vi "InitDrivebase.vi"   [LabVIEW 2019]
doc: "This VI initializes devices related directly to the drive subsystem."
uses:
  <vilib>/Rock Robotics/WPI/Solenoid/WPI_SolenoidChannel.ctl
  <vilib>/Rock Robotics/WPI/ThirdParty/Phoenix-LabVIEW/Motor Controller/Controls/CTRE_Phoenix_MotorControl_SupplyCurrentLimitConfiguration.ctl
  <vilib>/Rock Robotics/WPI/ThirdParty/Phoenix-LabVIEW/Motor Controller/Controls/CTRE_Phoenix_MotorControl_FeedbackDevice_TalonFX.ctl
  <vilib>/Rock Robotics/WPI/ThirdParty/Phoenix-LabVIEW/Motor Controller/Controls/CTRE_Phoenix_MotorControl_TalonFXInvertType.ctl
  <vilib>/Rock Robotics/WPI/ThirdParty/Phoenix-LabVIEW/Motor Controller/Controls/CTRE_Phoenix_MotorControl_NeutralMode.ctl
  <vilib>/Rock Robotics/WPI/Solenoid/WPI_SolenoidOpenDouble.vi
  refnums.vi
types:
  T1 = typedef "WPI_SolenoidChannel.ctl" = enum8{"Solenoid 0", "Solenoid 1", "Solenoid 2", "Solenoid 3", "Solenoid 4", "Solenoid 5", "Solenoid 6", "Solenoid 7", "Invalid"}
  T2 = typedef "CTRE_Phoenix_MotorControl_TalonFXInvertType.ctl" = enum16{"Counter-Clockwise", "Clockwise"}
  T3 = typedef "CTRE_Phoenix_MotorControl_FeedbackDevice_TalonFX.ctl" = i8
  T4 = typedef "CTRE_Phoenix_MotorControl_SupplyCurrentLimitConfiguration.ctl" = cluster{"Enable?":bool, "Current Limit":dbl, "Threshold Current":dbl, "Threshold Time":dbl}
  T5 = typedef "CTRE_Phoenix_MotorControl_NeutralMode.ctl" = enum8{"EEPROMSetting", "Override to Coast", "Override to Brake"}
  T6 = typedef "WPI_MotorControlDeviceRef.ctl" = cluster{"DeviceStatus":errorcluster, "Type":T7, "PWM":cluster{"PWM Channel":T8, "DeadBand":T9}, "CAN":cluster{"Device Number":u8, "SetOutput VI Ref":variant, "GetOutput VI Ref":variant, "Enable VI Ref":variant, "Disable VI Ref":variant, "Data":variant}, "Invert":bool, "DIO PWM":cluster{"PWM \"Enable\" Channel":T8, "DIOChannel":T10, "PWM Rate":dbl}}
  T7 = typedef "WPI_MotorControlType.ctl" = enum16{"PWM", "CAN", "DIO PWM"}
  T8 = typedef "FPGA_DIOPWMChannel.ctl" = enum8{"PWM 0", "PWM 1", "PWM 2", "PWM 3", "PWM 4", "PWM 5", "PWM 6", "PWM 7", "PWM 8", "PWM 9", "PWM MXP 0", "PWM MXP 1", "PWM MXP 2", "PWM MXP 3", "PWM MXP 4", "PWM MXP 5", "PWM MXP 6", "PWM MXP 7", "PWM MXP 8", "PWM MXP 9", "Invalid"}
  T9 = typedef "WPI_PWMDeadband.ctl" = cluster{"Name":string, "maxPositivePwm":i32, "minPositivePwm":i32, "centerPwm":i32, "maxNegativePwm":i32, "minNegativePwm":i32, "angularRange":u16}
  T10 = typedef "FPGA_DIOChannel.ctl" = enum8{"DIO 0", "DIO 1", "DIO 2", "DIO 3", "DIO 4", "DIO 5", "DIO 6", "DIO 7", "DIO 8", "DIO 9", "DIO MXP 0", "DIO MXP 1", "DIO MXP 2", "DIO MXP 3", "DIO MXP 4", "DIO MXP 5", "DIO MXP 6", "DIO MXP 7", "DIO MXP 8", "DIO MXP 9", "DIO MXP 10", "DIO MXP 11", "DIO MXP 12", "DIO MXP 13", "DIO MXP 14", "DIO MXP 15", "SPI Port CS1", "SPI Port CS2", "SPI Port CS3", "SPI Port MISO", "SPI Port MOSI", "Invalid"}
  T11 = typedef "WPI_SolenoidDevRef.ctl" = cluster{"DevStatus":errorcluster, "Pneumatics Control Module":u8, "Forward Solenoid Channel":T1, "Reverse Solenoid Channel":T1}
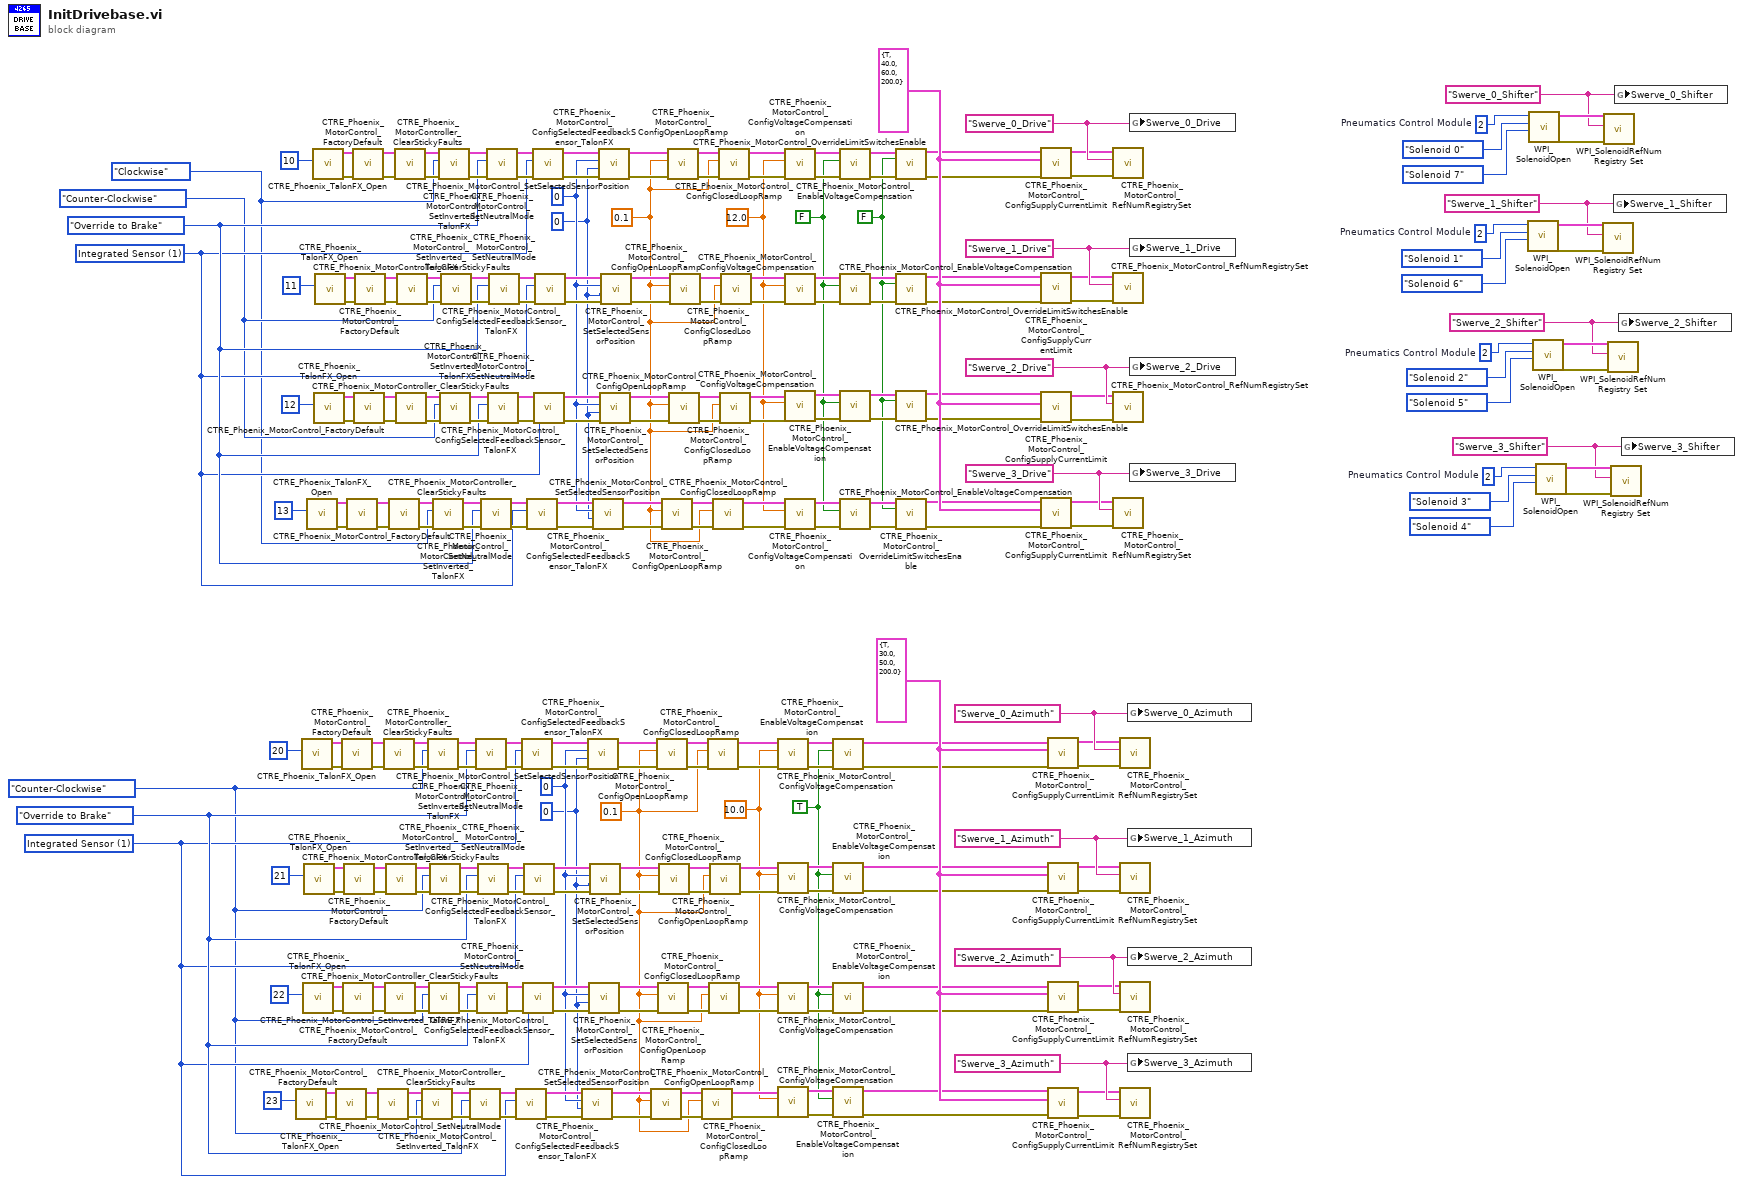
[diagram p0: block diagram]
diagram:
  w1 = FALSE ("Override Limit Switch Enable?")
  w19 = "Swerve_0_Shifter" ("refnum name")
  w24 = u8 2  # Pneumatics Control Module
  w25 = "Swerve_1_Shifter" ("refnum name")
  w30 = u8 2  # Pneumatics Control Module
  w31 = "Swerve_2_Shifter" ("refnum name")
  w36 = u8 2  # Pneumatics Control Module
  w37 = CTRE_Phoenix_MotorControl_TalonFXInvertType."Clockwise" ("Invert Type")
  w39 = TRUE ("Enable Voltage Compensation?")
  w40 = 10.0 ("Saturation Voltage")
  w41 = FALSE ("Enable Voltage Compensation?")
  w42 = 12.0 ("Saturation Voltage")
  w83 = T3 1 items=["Integrated Sensor"=1, "Sensor Sum (S0 + S1)"=9, "Sensor Difference (D0 - D1)"=10, "Remote Source 0"=11, "Remote Source 1"=12, "None"=14, "Software Emulated"=15] ("Talon FX Feedback Device")
  w88 = T4 {"Enable?"=TRUE, "Current Limit"=30.0, "Threshold Current"=50.0, "Threshold Time"=200.0} ("Supply Current Limit Configuration")
  w84 = 0.1 ("secondsFromNeutralToFull")
  w85 = u32 0 ("pidLoopIdx")
  w86 = 0 ("New Sensor Position")
  w87 = CTRE_Phoenix_MotorControl_NeutralMode."Override to Brake" ("Motor Control Neutral Mode")
  w18 = CTRE_Phoenix_MotorControl_TalonFXInvertType."Counter-Clockwise" ("Invert Type")
  w104 = "Swerve_0_Azimuth" ("refnum name")
  w124 = "Swerve_1_Azimuth" ("refnum name")
  w144 = "Swerve_2_Azimuth" ("refnum name")
  w164 = "Swerve_3_Azimuth" ("refnum name")
  w172 = T3 1 items=["Integrated Sensor"=1, "Sensor Sum (S0 + S1)"=9, "Sensor Difference (D0 - D1)"=10, "Remote Source 0"=11, "Remote Source 1"=12, "None"=14, "Software Emulated"=15] ("Talon FX Feedback Device")
  w174 = T4 {"Enable?"=TRUE, "Current Limit"=40.0, "Threshold Current"=60.0, "Threshold Time"=200.0} ("Supply Current Limit Configuration")
  w169 = 0.1 ("secondsFromNeutralToFull")
  w170 = u32 0 ("pidLoopIdx")
  w171 = 0 ("New Sensor Position")
  w173 = CTRE_Phoenix_MotorControl_NeutralMode."Override to Brake" ("Motor Control Neutral Mode")
  w38 = CTRE_Phoenix_MotorControl_TalonFXInvertType."Counter-Clockwise" ("Invert Type")
  w190 = "Swerve_0_Drive" ("refnum name")
  w210 = "Swerve_1_Drive" ("refnum name")
  w230 = "Swerve_2_Drive" ("refnum name")
  w250 = "Swerve_3_Drive" ("refnum name")
  w255 = "Swerve_3_Shifter" ("refnum name")
  w260 = u8 2  # Pneumatics Control Module
  n1 = call <vilib>:"CTRE_Phoenix_TalonFX_Open.vi"("Device Number"=u8 23 ("Drive 4L")) -> ("error out"=w153:errorcluster, "CAN Talon SRX Ref"=w160:T6)  [unwired: 9 in]
  n2 = call <vilib>:"CTRE_Phoenix_TalonFX_Open.vi"("Device Number"=u8 20 ("Drive 4L")) -> ("error out"=w93:errorcluster, "CAN Talon SRX Ref"=w100:T6)  [unwired: 9 in]
  n3 = call <vilib>:"CTRE_Phoenix_TalonFX_Open.vi"("Device Number"=u8 22 ("Drive 4L")) -> ("error out"=w133:errorcluster, "CAN Talon SRX Ref"=w140:T6)  [unwired: 9 in]
  n4 = call <vilib>:"CTRE_Phoenix_TalonFX_Open.vi"("Device Number"=u8 21 ("Drive 4L")) -> ("error out"=w113:errorcluster, "CAN Talon SRX Ref"=w120:T6)  [unwired: 9 in]
  n5 = call <vilib>:"CTRE_Phoenix_TalonFX_Open.vi"("Device Number"=u8 13 ("Drive 4L")) -> ("error out"=w239:errorcluster, "CAN Talon SRX Ref"=w246:T6)  [unwired: 9 in]
  n6 = call <vilib>:"CTRE_Phoenix_TalonFX_Open.vi"("Device Number"=u8 10 ("Drive 4L")) -> ("error out"=w179:errorcluster, "CAN Talon SRX Ref"=w186:T6)  [unwired: 9 in]
  n7 = call <vilib>:"CTRE_Phoenix_TalonFX_Open.vi"("Device Number"=u8 12 ("Drive 4L")) -> ("error out"=w219:errorcluster, "CAN Talon SRX Ref"=w226:T6)  [unwired: 9 in]
  n8 = call <vilib>:"CTRE_Phoenix_TalonFX_Open.vi"("Device Number"=u8 11 ("Drive 4L")) -> ("error out"=w199:errorcluster, "CAN Talon SRX Ref"=w206:T6)  [unwired: 9 in]
  n9 = call <vilib>:"CTRE_Phoenix_MotorControl_FactoryDefault.vi"("error in"=w153, "PhoenixMotorControlDevRef"=w160) -> ("error out"=w156:errorcluster, "PhoenixMotorControlDevRef"=w157:T6)  [unwired: 8 in]
  n10 = call <vilib>:"CTRE_Phoenix_MotorControl_FactoryDefault.vi"("error in"=w93, "PhoenixMotorControlDevRef"=w100) -> ("error out"=w96:errorcluster, "PhoenixMotorControlDevRef"=w97:T6)  [unwired: 8 in]
  n11 = call <vilib>:"CTRE_Phoenix_MotorControl_FactoryDefault.vi"("error in"=w133, "PhoenixMotorControlDevRef"=w140) -> ("error out"=w136:errorcluster, "PhoenixMotorControlDevRef"=w137:T6)  [unwired: 8 in]
  n12 = call <vilib>:"CTRE_Phoenix_MotorControl_FactoryDefault.vi"("error in"=w113, "PhoenixMotorControlDevRef"=w120) -> ("error out"=w116:errorcluster, "PhoenixMotorControlDevRef"=w117:T6)  [unwired: 8 in]
  n13 = call <vilib>:"CTRE_Phoenix_MotorControl_FactoryDefault.vi"("error in"=w239, "PhoenixMotorControlDevRef"=w246) -> ("error out"=w242:errorcluster, "PhoenixMotorControlDevRef"=w243:T6)  [unwired: 8 in]
  n14 = call <vilib>:"CTRE_Phoenix_MotorControl_FactoryDefault.vi"("error in"=w179, "PhoenixMotorControlDevRef"=w186) -> ("error out"=w182:errorcluster, "PhoenixMotorControlDevRef"=w183:T6)  [unwired: 8 in]
  n15 = call <vilib>:"CTRE_Phoenix_MotorControl_FactoryDefault.vi"("error in"=w219, "PhoenixMotorControlDevRef"=w226) -> ("error out"=w222:errorcluster, "PhoenixMotorControlDevRef"=w223:T6)  [unwired: 8 in]
  n16 = call <vilib>:"CTRE_Phoenix_MotorControl_FactoryDefault.vi"("error in"=w199, "PhoenixMotorControlDevRef"=w206) -> ("error out"=w202:errorcluster, "PhoenixMotorControlDevRef"=w203:T6)  [unwired: 8 in]
  n17 = call <vilib>:"CTRE_Phoenix_MotorController_ClearStickyFaults.vi"("error in"=w156, "PhoenixMotorControlDevRef"=w157) -> ("error out"=w155:errorcluster, "PhoenixMotorControlDevRef"=w154:T6)  [unwired: 8 in]
  n18 = call <vilib>:"CTRE_Phoenix_MotorController_ClearStickyFaults.vi"("error in"=w96, "PhoenixMotorControlDevRef"=w97) -> ("error out"=w95:errorcluster, "PhoenixMotorControlDevRef"=w94:T6)  [unwired: 8 in]
  n19 = call <vilib>:"CTRE_Phoenix_MotorController_ClearStickyFaults.vi"("error in"=w136, "PhoenixMotorControlDevRef"=w137) -> ("error out"=w135:errorcluster, "PhoenixMotorControlDevRef"=w134:T6)  [unwired: 8 in]
  n20 = call <vilib>:"CTRE_Phoenix_MotorController_ClearStickyFaults.vi"("error in"=w116, "PhoenixMotorControlDevRef"=w117) -> ("error out"=w115:errorcluster, "PhoenixMotorControlDevRef"=w114:T6)  [unwired: 8 in]
  n21 = call <vilib>:"CTRE_Phoenix_MotorController_ClearStickyFaults.vi"("error in"=w242, "PhoenixMotorControlDevRef"=w243) -> ("error out"=w241:errorcluster, "PhoenixMotorControlDevRef"=w240:T6)  [unwired: 8 in]
  n22 = call <vilib>:"CTRE_Phoenix_MotorController_ClearStickyFaults.vi"("error in"=w182, "PhoenixMotorControlDevRef"=w183) -> ("error out"=w181:errorcluster, "PhoenixMotorControlDevRef"=w180:T6)  [unwired: 8 in]
  n23 = call <vilib>:"CTRE_Phoenix_MotorController_ClearStickyFaults.vi"("error in"=w222, "PhoenixMotorControlDevRef"=w223) -> ("error out"=w221:errorcluster, "PhoenixMotorControlDevRef"=w220:T6)  [unwired: 8 in]
  n24 = call <vilib>:"CTRE_Phoenix_MotorController_ClearStickyFaults.vi"("error in"=w202, "PhoenixMotorControlDevRef"=w203) -> ("error out"=w201:errorcluster, "PhoenixMotorControlDevRef"=w200:T6)  [unwired: 8 in]
  n25 = call <vilib>:"CTRE_Phoenix_MotorControl_SetInverted_TalonFX.vi"("error in (no error)"=w155, "Invert Type"=w18, "PhoenixMotorControlDevRef"=w154) -> ("error out"=w167:errorcluster, "PhoenixMotorControlDevRef"=w168:T6)  [unwired: 7 in]
  n26 = call <vilib>:"CTRE_Phoenix_MotorControl_SetInverted_TalonFX.vi"("error in (no error)"=w95, "Invert Type"=w18, "PhoenixMotorControlDevRef"=w94) -> ("error out"=w107:errorcluster, "PhoenixMotorControlDevRef"=w108:T6)  [unwired: 7 in]
  n27 = call <vilib>:"CTRE_Phoenix_MotorControl_SetInverted_TalonFX.vi"("error in (no error)"=w135, "Invert Type"=w18, "PhoenixMotorControlDevRef"=w134) -> ("error out"=w147:errorcluster, "PhoenixMotorControlDevRef"=w148:T6)  [unwired: 7 in]
  n28 = call <vilib>:"CTRE_Phoenix_MotorControl_SetInverted_TalonFX.vi"("error in (no error)"=w115, "Invert Type"=w18, "PhoenixMotorControlDevRef"=w114) -> ("error out"=w127:errorcluster, "PhoenixMotorControlDevRef"=w128:T6)  [unwired: 7 in]
  n29 = call <vilib>:"CTRE_Phoenix_MotorControl_SetInverted_TalonFX.vi"("error in (no error)"=w241, "Invert Type"=w37, "PhoenixMotorControlDevRef"=w240) -> ("error out"=w253:errorcluster, "PhoenixMotorControlDevRef"=w254:T6)  [unwired: 7 in]
  n30 = call <vilib>:"CTRE_Phoenix_MotorControl_SetInverted_TalonFX.vi"("error in (no error)"=w181, "Invert Type"=w37, "PhoenixMotorControlDevRef"=w180) -> ("error out"=w193:errorcluster, "PhoenixMotorControlDevRef"=w194:T6)  [unwired: 7 in]
  n31 = call <vilib>:"CTRE_Phoenix_MotorControl_SetInverted_TalonFX.vi"("error in (no error)"=w221, "Invert Type"=w38, "PhoenixMotorControlDevRef"=w220) -> ("error out"=w233:errorcluster, "PhoenixMotorControlDevRef"=w234:T6)  [unwired: 7 in]
  n32 = call <vilib>:"CTRE_Phoenix_MotorControl_SetInverted_TalonFX.vi"("error in (no error)"=w201, "Invert Type"=w38, "PhoenixMotorControlDevRef"=w200) -> ("error out"=w213:errorcluster, "PhoenixMotorControlDevRef"=w214:T6)  [unwired: 7 in]
  n33 = call <vilib>:"CTRE_Phoenix_MotorControl_SetNeutralMode.vi"("error in (no error)"=w167, "Motor Control Neutral Mode"=w87, "PhoenixMotorControlDevRef"=w168) -> ("error out"=w151:errorcluster, "PhoenixMotorControlDevRef"=w152:T6)  [unwired: 7 in]
  n34 = call <vilib>:"CTRE_Phoenix_MotorControl_SetNeutralMode.vi"("error in (no error)"=w107, "Motor Control Neutral Mode"=w87, "PhoenixMotorControlDevRef"=w108) -> ("error out"=w91:errorcluster, "PhoenixMotorControlDevRef"=w92:T6)  [unwired: 7 in]
  n35 = call <vilib>:"CTRE_Phoenix_MotorControl_SetNeutralMode.vi"("error in (no error)"=w147, "Motor Control Neutral Mode"=w87, "PhoenixMotorControlDevRef"=w148) -> ("error out"=w131:errorcluster, "PhoenixMotorControlDevRef"=w132:T6)  [unwired: 7 in]
  n36 = call <vilib>:"CTRE_Phoenix_MotorControl_SetNeutralMode.vi"("error in (no error)"=w127, "Motor Control Neutral Mode"=w87, "PhoenixMotorControlDevRef"=w128) -> ("error out"=w111:errorcluster, "PhoenixMotorControlDevRef"=w112:T6)  [unwired: 7 in]
  n37 = call <vilib>:"CTRE_Phoenix_MotorControl_SetNeutralMode.vi"("error in (no error)"=w253, "Motor Control Neutral Mode"=w173, "PhoenixMotorControlDevRef"=w254) -> ("error out"=w237:errorcluster, "PhoenixMotorControlDevRef"=w238:T6)  [unwired: 7 in]
  n38 = call <vilib>:"CTRE_Phoenix_MotorControl_SetNeutralMode.vi"("error in (no error)"=w193, "Motor Control Neutral Mode"=w173, "PhoenixMotorControlDevRef"=w194) -> ("error out"=w177:errorcluster, "PhoenixMotorControlDevRef"=w178:T6)  [unwired: 7 in]
  n39 = call <vilib>:"CTRE_Phoenix_MotorControl_SetNeutralMode.vi"("error in (no error)"=w233, "Motor Control Neutral Mode"=w173, "PhoenixMotorControlDevRef"=w234) -> ("error out"=w217:errorcluster, "PhoenixMotorControlDevRef"=w218:T6)  [unwired: 7 in]
  n40 = call <vilib>:"CTRE_Phoenix_MotorControl_SetNeutralMode.vi"("error in (no error)"=w213, "Motor Control Neutral Mode"=w173, "PhoenixMotorControlDevRef"=w214) -> ("error out"=w197:errorcluster, "PhoenixMotorControlDevRef"=w198:T6)  [unwired: 7 in]
  n41 = call <vilib>:"CTRE_Phoenix_MotorControl_ConfigSelectedFeedbackSensor_TalonFX.vi"("error in (no error)"=w151, "Talon FX Feedback Device"=w83, "PhoenixMotorControlDevRef"=w152) -> ("error out"=w149:errorcluster, "PhoenixMotorControlDevRef"=w150:T6)  [unwired: 7 in]
  n42 = call <vilib>:"CTRE_Phoenix_MotorControl_ConfigSelectedFeedbackSensor_TalonFX.vi"("error in (no error)"=w91, "Talon FX Feedback Device"=w83, "PhoenixMotorControlDevRef"=w92) -> ("error out"=w89:errorcluster, "PhoenixMotorControlDevRef"=w90:T6)  [unwired: 7 in]
  n43 = call <vilib>:"CTRE_Phoenix_MotorControl_ConfigSelectedFeedbackSensor_TalonFX.vi"("error in (no error)"=w131, "Talon FX Feedback Device"=w83, "PhoenixMotorControlDevRef"=w132) -> ("error out"=w129:errorcluster, "PhoenixMotorControlDevRef"=w130:T6)  [unwired: 7 in]
  n44 = call <vilib>:"CTRE_Phoenix_MotorControl_ConfigSelectedFeedbackSensor_TalonFX.vi"("error in (no error)"=w111, "Talon FX Feedback Device"=w83, "PhoenixMotorControlDevRef"=w112) -> ("error out"=w109:errorcluster, "PhoenixMotorControlDevRef"=w110:T6)  [unwired: 7 in]
  n45 = call <vilib>:"CTRE_Phoenix_MotorControl_ConfigSelectedFeedbackSensor_TalonFX.vi"("error in (no error)"=w237, "Talon FX Feedback Device"=w172, "PhoenixMotorControlDevRef"=w238) -> ("error out"=w235:errorcluster, "PhoenixMotorControlDevRef"=w236:T6)  [unwired: 7 in]
  n46 = call <vilib>:"CTRE_Phoenix_MotorControl_ConfigSelectedFeedbackSensor_TalonFX.vi"("error in (no error)"=w177, "Talon FX Feedback Device"=w172, "PhoenixMotorControlDevRef"=w178) -> ("error out"=w175:errorcluster, "PhoenixMotorControlDevRef"=w176:T6)  [unwired: 7 in]
  n47 = call <vilib>:"CTRE_Phoenix_MotorControl_ConfigSelectedFeedbackSensor_TalonFX.vi"("error in (no error)"=w217, "Talon FX Feedback Device"=w172, "PhoenixMotorControlDevRef"=w218) -> ("error out"=w215:errorcluster, "PhoenixMotorControlDevRef"=w216:T6)  [unwired: 7 in]
  n48 = call <vilib>:"CTRE_Phoenix_MotorControl_ConfigSelectedFeedbackSensor_TalonFX.vi"("error in (no error)"=w197, "Talon FX Feedback Device"=w172, "PhoenixMotorControlDevRef"=w198) -> ("error out"=w195:errorcluster, "PhoenixMotorControlDevRef"=w196:T6)  [unwired: 7 in]
  n49 = call <vilib>:"CTRE_Phoenix_MotorControl_SetSelectedSensorPosition.vi"("error in (no error)"=w149, "pidLoopIdx"=w85, "New Sensor Position"=w86, "PhoenixMotorControlDevRef"=w150) -> ("error out"=w166:errorcluster, "PhoenixMotorControlDevRef"=w165:T6)  [unwired: 6 in]
  n50 = call <vilib>:"CTRE_Phoenix_MotorControl_SetSelectedSensorPosition.vi"("error in (no error)"=w89, "pidLoopIdx"=w85, "New Sensor Position"=w86, "PhoenixMotorControlDevRef"=w90) -> ("error out"=w106:errorcluster, "PhoenixMotorControlDevRef"=w105:T6)  [unwired: 6 in]
  n51 = call <vilib>:"CTRE_Phoenix_MotorControl_SetSelectedSensorPosition.vi"("error in (no error)"=w129, "pidLoopIdx"=w85, "New Sensor Position"=w86, "PhoenixMotorControlDevRef"=w130) -> ("error out"=w146:errorcluster, "PhoenixMotorControlDevRef"=w145:T6)  [unwired: 6 in]
  n52 = call <vilib>:"CTRE_Phoenix_MotorControl_SetSelectedSensorPosition.vi"("error in (no error)"=w109, "pidLoopIdx"=w85, "New Sensor Position"=w86, "PhoenixMotorControlDevRef"=w110) -> ("error out"=w126:errorcluster, "PhoenixMotorControlDevRef"=w125:T6)  [unwired: 6 in]
  n53 = call <vilib>:"CTRE_Phoenix_MotorControl_SetSelectedSensorPosition.vi"("error in (no error)"=w235, "pidLoopIdx"=w170, "New Sensor Position"=w171, "PhoenixMotorControlDevRef"=w236) -> ("error out"=w252:errorcluster, "PhoenixMotorControlDevRef"=w251:T6)  [unwired: 6 in]
  n54 = call <vilib>:"CTRE_Phoenix_MotorControl_SetSelectedSensorPosition.vi"("error in (no error)"=w175, "pidLoopIdx"=w170, "New Sensor Position"=w171, "PhoenixMotorControlDevRef"=w176) -> ("error out"=w192:errorcluster, "PhoenixMotorControlDevRef"=w191:T6)  [unwired: 6 in]
  n55 = call <vilib>:"CTRE_Phoenix_MotorControl_SetSelectedSensorPosition.vi"("error in (no error)"=w215, "pidLoopIdx"=w170, "New Sensor Position"=w171, "PhoenixMotorControlDevRef"=w216) -> ("error out"=w232:errorcluster, "PhoenixMotorControlDevRef"=w231:T6)  [unwired: 6 in]
  n56 = call <vilib>:"CTRE_Phoenix_MotorControl_SetSelectedSensorPosition.vi"("error in (no error)"=w195, "pidLoopIdx"=w170, "New Sensor Position"=w171, "PhoenixMotorControlDevRef"=w196) -> ("error out"=w212:errorcluster, "PhoenixMotorControlDevRef"=w211:T6)  [unwired: 6 in]
  n57 = call <vilib>:"CTRE_Phoenix_MotorControl_ConfigOpenLoopRamp.vi"("error in (no error)"=w166, "secondsFromNeutralToFull"=w84, "PhoenixMotorControlDevRef"=w165) -> ("error out"=w158:errorcluster, "PhoenixMotorControlDevRef"=w159:T6)  [unwired: 7 in]
  n58 = call <vilib>:"CTRE_Phoenix_MotorControl_ConfigOpenLoopRamp.vi"("error in (no error)"=w106, "secondsFromNeutralToFull"=w84, "PhoenixMotorControlDevRef"=w105) -> ("error out"=w98:errorcluster, "PhoenixMotorControlDevRef"=w99:T6)  [unwired: 7 in]
  n59 = call <vilib>:"CTRE_Phoenix_MotorControl_ConfigOpenLoopRamp.vi"("error in (no error)"=w146, "secondsFromNeutralToFull"=w84, "PhoenixMotorControlDevRef"=w145) -> ("error out"=w138:errorcluster, "PhoenixMotorControlDevRef"=w139:T6)  [unwired: 7 in]
  n60 = call <vilib>:"CTRE_Phoenix_MotorControl_ConfigOpenLoopRamp.vi"("error in (no error)"=w126, "secondsFromNeutralToFull"=w84, "PhoenixMotorControlDevRef"=w125) -> ("error out"=w118:errorcluster, "PhoenixMotorControlDevRef"=w119:T6)  [unwired: 7 in]
  n61 = call <vilib>:"CTRE_Phoenix_MotorControl_ConfigOpenLoopRamp.vi"("error in (no error)"=w252, "secondsFromNeutralToFull"=w169, "PhoenixMotorControlDevRef"=w251) -> ("error out"=w244:errorcluster, "PhoenixMotorControlDevRef"=w245:T6)  [unwired: 7 in]
  n62 = call <vilib>:"CTRE_Phoenix_MotorControl_ConfigOpenLoopRamp.vi"("error in (no error)"=w192, "secondsFromNeutralToFull"=w169, "PhoenixMotorControlDevRef"=w191) -> ("error out"=w184:errorcluster, "PhoenixMotorControlDevRef"=w185:T6)  [unwired: 7 in]
  n63 = call <vilib>:"CTRE_Phoenix_MotorControl_ConfigOpenLoopRamp.vi"("error in (no error)"=w232, "secondsFromNeutralToFull"=w169, "PhoenixMotorControlDevRef"=w231) -> ("error out"=w224:errorcluster, "PhoenixMotorControlDevRef"=w225:T6)  [unwired: 7 in]
  n64 = call <vilib>:"CTRE_Phoenix_MotorControl_ConfigOpenLoopRamp.vi"("error in (no error)"=w212, "secondsFromNeutralToFull"=w169, "PhoenixMotorControlDevRef"=w211) -> ("error out"=w204:errorcluster, "PhoenixMotorControlDevRef"=w205:T6)  [unwired: 7 in]
  n65 = call <vilib>:"CTRE_Phoenix_MotorControl_ConfigClosedLoopRamp.vi"("error in (no error)"=w158, "secondsFromNeutralToFull"=w84, "PhoenixMotorControlDevRef"=w159) -> ("error out"=w45:errorcluster, "PhoenixMotorControlDevRef"=w46:T6)  [unwired: 7 in]
  n66 = call <vilib>:"CTRE_Phoenix_MotorControl_ConfigClosedLoopRamp.vi"("error in (no error)"=w98, "secondsFromNeutralToFull"=w84, "PhoenixMotorControlDevRef"=w99) -> ("error out"=w57:errorcluster, "PhoenixMotorControlDevRef"=w58:T6)  [unwired: 7 in]
  n67 = call <vilib>:"CTRE_Phoenix_MotorControl_ConfigClosedLoopRamp.vi"("error in (no error)"=w138, "secondsFromNeutralToFull"=w84, "PhoenixMotorControlDevRef"=w139) -> ("error out"=w49:errorcluster, "PhoenixMotorControlDevRef"=w50:T6)  [unwired: 7 in]
  n68 = call <vilib>:"CTRE_Phoenix_MotorControl_ConfigClosedLoopRamp.vi"("error in (no error)"=w118, "secondsFromNeutralToFull"=w84, "PhoenixMotorControlDevRef"=w119) -> ("error out"=w53:errorcluster, "PhoenixMotorControlDevRef"=w54:T6)  [unwired: 7 in]
  n69 = call <vilib>:"CTRE_Phoenix_MotorControl_ConfigClosedLoopRamp.vi"("error in (no error)"=w244, "secondsFromNeutralToFull"=w169, "PhoenixMotorControlDevRef"=w245) -> ("error out"=w59:errorcluster, "PhoenixMotorControlDevRef"=w60:T6)  [unwired: 7 in]
  n70 = call <vilib>:"CTRE_Phoenix_MotorControl_ConfigClosedLoopRamp.vi"("error in (no error)"=w184, "secondsFromNeutralToFull"=w169, "PhoenixMotorControlDevRef"=w185) -> ("error out"=w65:errorcluster, "PhoenixMotorControlDevRef"=w66:T6)  [unwired: 7 in]
  n71 = call <vilib>:"CTRE_Phoenix_MotorControl_ConfigClosedLoopRamp.vi"("error in (no error)"=w224, "secondsFromNeutralToFull"=w169, "PhoenixMotorControlDevRef"=w225) -> ("error out"=w61:errorcluster, "PhoenixMotorControlDevRef"=w62:T6)  [unwired: 7 in]
  n72 = call <vilib>:"CTRE_Phoenix_MotorControl_ConfigClosedLoopRamp.vi"("error in (no error)"=w204, "secondsFromNeutralToFull"=w169, "PhoenixMotorControlDevRef"=w205) -> ("error out"=w63:errorcluster, "PhoenixMotorControlDevRef"=w64:T6)  [unwired: 7 in]
  n73 = call <vilib>:"CTRE_Phoenix_MotorControl_ConfigVoltageCompensation.vi"("error in (no error)"=w57, "Saturation Voltage"=w40, "PhoenixMotorControlDevRef"=w58) -> ("error out"=w73:errorcluster, "PhoenixMotorControlDevRef"=w74:T6)  [unwired: 7 in]
  n74 = call <vilib>:"CTRE_Phoenix_MotorControl_ConfigVoltageCompensation.vi"("error in (no error)"=w53, "Saturation Voltage"=w40, "PhoenixMotorControlDevRef"=w54) -> ("error out"=w71:errorcluster, "PhoenixMotorControlDevRef"=w72:T6)  [unwired: 7 in]
  n75 = call <vilib>:"CTRE_Phoenix_MotorControl_ConfigVoltageCompensation.vi"("error in (no error)"=w49, "Saturation Voltage"=w40, "PhoenixMotorControlDevRef"=w50) -> ("error out"=w69:errorcluster, "PhoenixMotorControlDevRef"=w70:T6)  [unwired: 7 in]
  n76 = call <vilib>:"CTRE_Phoenix_MotorControl_ConfigVoltageCompensation.vi"("error in (no error)"=w45, "Saturation Voltage"=w40, "PhoenixMotorControlDevRef"=w46) -> ("error out"=w67:errorcluster, "PhoenixMotorControlDevRef"=w68:T6)  [unwired: 7 in]
  n77 = call <vilib>:"CTRE_Phoenix_MotorControl_ConfigVoltageCompensation.vi"("error in (no error)"=w65, "Saturation Voltage"=w42, "PhoenixMotorControlDevRef"=w66) -> ("error out"=w81:errorcluster, "PhoenixMotorControlDevRef"=w82:T6)  [unwired: 7 in]
  n78 = call <vilib>:"CTRE_Phoenix_MotorControl_ConfigVoltageCompensation.vi"("error in (no error)"=w63, "Saturation Voltage"=w42, "PhoenixMotorControlDevRef"=w64) -> ("error out"=w79:errorcluster, "PhoenixMotorControlDevRef"=w80:T6)  [unwired: 7 in]
  n79 = call <vilib>:"CTRE_Phoenix_MotorControl_ConfigVoltageCompensation.vi"("error in (no error)"=w61, "Saturation Voltage"=w42, "PhoenixMotorControlDevRef"=w62) -> ("error out"=w77:errorcluster, "PhoenixMotorControlDevRef"=w78:T6)  [unwired: 7 in]
  n80 = call <vilib>:"CTRE_Phoenix_MotorControl_ConfigVoltageCompensation.vi"("error in (no error)"=w59, "Saturation Voltage"=w42, "PhoenixMotorControlDevRef"=w60) -> ("error out"=w75:errorcluster, "PhoenixMotorControlDevRef"=w76:T6)  [unwired: 7 in]
  n81 = call <vilib>:"CTRE_Phoenix_MotorControl_EnableVoltageCompensation.vi"("error in (no error)"=w73, "Enable Voltage Compensation?"=w39, "PhoenixMotorControlDevRef"=w74) -> ("error out"=w55:errorcluster, "PhoenixMotorControlDevRef"=w56:T6)  [unwired: 7 in]
  n82 = call <vilib>:"CTRE_Phoenix_MotorControl_EnableVoltageCompensation.vi"("error in (no error)"=w71, "Enable Voltage Compensation?"=w39, "PhoenixMotorControlDevRef"=w72) -> ("error out"=w51:errorcluster, "PhoenixMotorControlDevRef"=w52:T6)  [unwired: 7 in]
  n83 = call <vilib>:"CTRE_Phoenix_MotorControl_EnableVoltageCompensation.vi"("error in (no error)"=w69, "Enable Voltage Compensation?"=w39, "PhoenixMotorControlDevRef"=w70) -> ("error out"=w47:errorcluster, "PhoenixMotorControlDevRef"=w48:T6)  [unwired: 7 in]
  n84 = call <vilib>:"CTRE_Phoenix_MotorControl_EnableVoltageCompensation.vi"("error in (no error)"=w67, "Enable Voltage Compensation?"=w39, "PhoenixMotorControlDevRef"=w68) -> ("error out"=w43:errorcluster, "PhoenixMotorControlDevRef"=w44:T6)  [unwired: 7 in]
  n85 = call <vilib>:"CTRE_Phoenix_MotorControl_EnableVoltageCompensation.vi"("error in (no error)"=w81, "Enable Voltage Compensation?"=w41, "PhoenixMotorControlDevRef"=w82) -> ("error out"=w16:errorcluster, "PhoenixMotorControlDevRef"=w17:T6)  [unwired: 7 in]
  n86 = call <vilib>:"CTRE_Phoenix_MotorControl_EnableVoltageCompensation.vi"("error in (no error)"=w79, "Enable Voltage Compensation?"=w41, "PhoenixMotorControlDevRef"=w80) -> ("error out"=w14:errorcluster, "PhoenixMotorControlDevRef"=w15:T6)  [unwired: 7 in]
  n87 = call <vilib>:"CTRE_Phoenix_MotorControl_EnableVoltageCompensation.vi"("error in (no error)"=w77, "Enable Voltage Compensation?"=w41, "PhoenixMotorControlDevRef"=w78) -> ("error out"=w12:errorcluster, "PhoenixMotorControlDevRef"=w13:T6)  [unwired: 7 in]
  n88 = call <vilib>:"CTRE_Phoenix_MotorControl_EnableVoltageCompensation.vi"("error in (no error)"=w75, "Enable Voltage Compensation?"=w41, "PhoenixMotorControlDevRef"=w76) -> ("error out"=w10:errorcluster, "PhoenixMotorControlDevRef"=w11:T6)  [unwired: 7 in]
  n89 = call <vilib>:"CTRE_Phoenix_MotorControl_OverrideLimitSwitchesEnable.vi"("PhoenixMotorControlDevRef"=w17, "Override Limit Switch Enable?"=w1, "error in (no error)"=w16) -> ("PhoenixMotorControlDevRef"=w9:T6, "error out"=w8:errorcluster)  [unwired: 11 in]
  n90 = call <vilib>:"CTRE_Phoenix_MotorControl_OverrideLimitSwitchesEnable.vi"("PhoenixMotorControlDevRef"=w15, "Override Limit Switch Enable?"=w1, "error in (no error)"=w14) -> ("PhoenixMotorControlDevRef"=w7:T6, "error out"=w6:errorcluster)  [unwired: 11 in]
  n91 = call <vilib>:"CTRE_Phoenix_MotorControl_OverrideLimitSwitchesEnable.vi"("PhoenixMotorControlDevRef"=w13, "Override Limit Switch Enable?"=w1, "error in (no error)"=w12) -> ("PhoenixMotorControlDevRef"=w5:T6, "error out"=w4:errorcluster)  [unwired: 11 in]
  n92 = call <vilib>:"CTRE_Phoenix_MotorControl_OverrideLimitSwitchesEnable.vi"("PhoenixMotorControlDevRef"=w11, "Override Limit Switch Enable?"=w1, "error in (no error)"=w10) -> ("PhoenixMotorControlDevRef"=w3:T6, "error out"=w2:errorcluster)  [unwired: 11 in]
  n93 = call <vilib>:"CTRE_Phoenix_MotorControl_ConfigSupplyCurrentLimit.vi"("error in (no error)"=w8, "Supply Current Limit Configuration"=w174, "PhoenixMotorControlDevRef"=w9) -> ("error out"=w188:errorcluster, "PhoenixMotorControlDevRef"=w189:T6)  [unwired: 7 in]
  n94 = call <vilib>:"CTRE_Phoenix_MotorControl_ConfigSupplyCurrentLimit.vi"("error in (no error)"=w6, "Supply Current Limit Configuration"=w174, "PhoenixMotorControlDevRef"=w7) -> ("error out"=w208:errorcluster, "PhoenixMotorControlDevRef"=w209:T6)  [unwired: 7 in]
  n95 = call <vilib>:"CTRE_Phoenix_MotorControl_ConfigSupplyCurrentLimit.vi"("error in (no error)"=w4, "Supply Current Limit Configuration"=w174, "PhoenixMotorControlDevRef"=w5) -> ("error out"=w228:errorcluster, "PhoenixMotorControlDevRef"=w229:T6)  [unwired: 7 in]
  n96 = call <vilib>:"CTRE_Phoenix_MotorControl_ConfigSupplyCurrentLimit.vi"("error in (no error)"=w2, "Supply Current Limit Configuration"=w174, "PhoenixMotorControlDevRef"=w3) -> ("error out"=w248:errorcluster, "PhoenixMotorControlDevRef"=w249:T6)  [unwired: 7 in]
  n97 = call <vilib>:"CTRE_Phoenix_MotorControl_ConfigSupplyCurrentLimit.vi"("error in (no error)"=w55, "Supply Current Limit Configuration"=w88, "PhoenixMotorControlDevRef"=w56) -> ("error out"=w102:errorcluster, "PhoenixMotorControlDevRef"=w103:T6)  [unwired: 7 in]
  n98 = call <vilib>:"CTRE_Phoenix_MotorControl_ConfigSupplyCurrentLimit.vi"("error in (no error)"=w51, "Supply Current Limit Configuration"=w88, "PhoenixMotorControlDevRef"=w52) -> ("error out"=w122:errorcluster, "PhoenixMotorControlDevRef"=w123:T6)  [unwired: 7 in]
  n99 = call <vilib>:"CTRE_Phoenix_MotorControl_ConfigSupplyCurrentLimit.vi"("error in (no error)"=w47, "Supply Current Limit Configuration"=w88, "PhoenixMotorControlDevRef"=w48) -> ("error out"=w142:errorcluster, "PhoenixMotorControlDevRef"=w143:T6)  [unwired: 7 in]
  n100 = call <vilib>:"CTRE_Phoenix_MotorControl_ConfigSupplyCurrentLimit.vi"("error in (no error)"=w43, "Supply Current Limit Configuration"=w88, "PhoenixMotorControlDevRef"=w44) -> ("error out"=w162:errorcluster, "PhoenixMotorControlDevRef"=w163:T6)  [unwired: 7 in]
  n101 = call <vilib>:"CTRE_Phoenix_MotorControl_RefNumRegistrySet.vi"("error in (no error)"=w188, "refnum name"=w190, "PhoenixMotorControlDevRef"=w189) -> ()  [unwired: 7 in, 2 out]
  n102 = call <vilib>:"CTRE_Phoenix_MotorControl_RefNumRegistrySet.vi"("error in (no error)"=w208, "refnum name"=w210, "PhoenixMotorControlDevRef"=w209) -> ()  [unwired: 7 in, 2 out]
  n103 = call <vilib>:"CTRE_Phoenix_MotorControl_RefNumRegistrySet.vi"("error in (no error)"=w228, "refnum name"=w230, "PhoenixMotorControlDevRef"=w229) -> ()  [unwired: 7 in, 2 out]
  n104 = call <vilib>:"CTRE_Phoenix_MotorControl_RefNumRegistrySet.vi"("error in (no error)"=w248, "refnum name"=w250, "PhoenixMotorControlDevRef"=w249) -> ()  [unwired: 7 in, 2 out]
  n105 = call <vilib>:"CTRE_Phoenix_MotorControl_RefNumRegistrySet.vi"("error in (no error)"=w102, "refnum name"=w104, "PhoenixMotorControlDevRef"=w103) -> ()  [unwired: 7 in, 2 out]
  n106 = call <vilib>:"CTRE_Phoenix_MotorControl_RefNumRegistrySet.vi"("error in (no error)"=w122, "refnum name"=w124, "PhoenixMotorControlDevRef"=w123) -> ()  [unwired: 7 in, 2 out]
  n107 = call <vilib>:"CTRE_Phoenix_MotorControl_RefNumRegistrySet.vi"("error in (no error)"=w142, "refnum name"=w144, "PhoenixMotorControlDevRef"=w143) -> ()  [unwired: 7 in, 2 out]
  n108 = call <vilib>:"CTRE_Phoenix_MotorControl_RefNumRegistrySet.vi"("error in (no error)"=w162, "refnum name"=w164, "PhoenixMotorControlDevRef"=w163) -> ()  [unwired: 7 in, 2 out]
  n109 = global write "refnums.vi" "Swerve_0_Azimuth"(w104) -> ()
  n110 = global write "refnums.vi" "Swerve_1_Azimuth"(w124) -> ()
  n111 = global write "refnums.vi" "Swerve_2_Azimuth"(w144) -> ()
  n112 = global write "refnums.vi" "Swerve_3_Azimuth"(w164) -> ()
  n113 = global write "refnums.vi" "Swerve_0_Drive"(w190) -> ()
  n114 = global write "refnums.vi" "Swerve_1_Drive"(w210) -> ()
  n115 = global write "refnums.vi" "Swerve_2_Drive"(w230) -> ()
  n116 = global write "refnums.vi" "Swerve_3_Drive"(w250) -> ()
  n117 = call-poly <vilib>:"WPI_SolenoidOpen.vi"("Reverse Solenoid Channel"=WPI_SolenoidChannel."Solenoid 6", "Forward Solenoid Channel"=WPI_SolenoidChannel."Solenoid 1", "Pneumatics Control Module (0)"=w30) -> ("error out"=w26:errorcluster, "SolenoidDevRef"=w27:T11)  [unwired: 7 in]
  n118 = call-poly <vilib>:"WPI_SolenoidOpen.vi"("Reverse Solenoid Channel"=WPI_SolenoidChannel."Solenoid 7", "Forward Solenoid Channel"=WPI_SolenoidChannel."Solenoid 0", "Pneumatics Control Module (0)"=w24) -> ("error out"=w20:errorcluster, "SolenoidDevRef"=w21:T11)  [unwired: 7 in]
  n119 = call-poly <vilib>:"WPI_SolenoidOpen.vi"("Reverse Solenoid Channel"=WPI_SolenoidChannel."Solenoid 5", "Forward Solenoid Channel"=WPI_SolenoidChannel."Solenoid 2", "Pneumatics Control Module (0)"=w36) -> ("error out"=w32:errorcluster, "SolenoidDevRef"=w33:T11)  [unwired: 7 in]
  n120 = call-poly <vilib>:"WPI_SolenoidOpen.vi"("Reverse Solenoid Channel"=WPI_SolenoidChannel."Solenoid 4", "Forward Solenoid Channel"=WPI_SolenoidChannel."Solenoid 3", "Pneumatics Control Module (0)"=w260) -> ("error out"=w256:errorcluster, "SolenoidDevRef"=w257:T11)  [unwired: 7 in]
  n121 = call <vilib>:"WPI_SolenoidRefNum Registry Set.vi"("error in (no error)"=w26, "refnum name"=w25, "SolenoidDevRef"=w27) -> ()  [unwired: 7 in, 2 out]
  n122 = call <vilib>:"WPI_SolenoidRefNum Registry Set.vi"("error in (no error)"=w20, "refnum name"=w19, "SolenoidDevRef"=w21) -> ()  [unwired: 7 in, 2 out]
  n123 = call <vilib>:"WPI_SolenoidRefNum Registry Set.vi"("error in (no error)"=w32, "refnum name"=w31, "SolenoidDevRef"=w33) -> ()  [unwired: 7 in, 2 out]
  n124 = call <vilib>:"WPI_SolenoidRefNum Registry Set.vi"("error in (no error)"=w256, "refnum name"=w255, "SolenoidDevRef"=w257) -> ()  [unwired: 7 in, 2 out]
  n125 = global write "refnums.vi" "Swerve_1_Shifter"(w25) -> ()
  n126 = global write "refnums.vi" "Swerve_0_Shifter"(w19) -> ()
  n127 = global write "refnums.vi" "Swerve_2_Shifter"(w31) -> ()
  n128 = global write "refnums.vi" "Swerve_3_Shifter"(w255) -> ()
